vi "TEST.vi"(5 "Scaling":dbl, 6 "#":i32) -> (1 "Array":dbl[](array[numeric]))   [LabVIEW 2014]
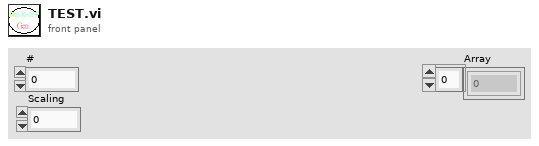
[diagram p1: front panel]
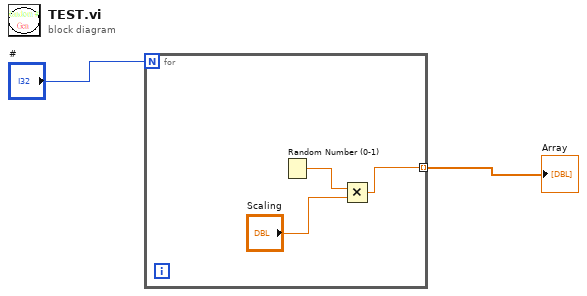
[diagram p0: block diagram]
diagram:
  n1 = for {
    N: "#" -> [_]
    tunnel: [w3] -> w2 mode=indexing
    n2 = Random Number (0-1)() -> (number: 0 to 1=w5:dbl)
    n3 = Multiply(x=w5, y="Scaling") -> (x*y=w3:dbl)
  }
  "Array" <- w2
